vi "Overlay circle modified.vi"(0 "Image In":T1, 1 "Measurment Name":string, 2 "Overlay width":i32, 3 "Overlay color":u32(colorbox), 4 "Circle center":T2, 5 "error in (no error)":errorcluster) -> (14 "Image out":T1, 19 "error out":errorcluster)   [LabVIEW 2019]
uses:
  <vilib>/vision/Image Controls.llb/IMAQ Image.ctl
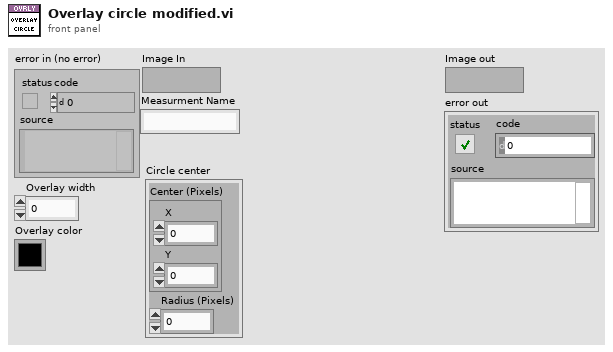
[diagram p1: front panel]
types:
  T1 = typedef "IMAQ Image.ctl" = refnum<image>
  T2 = cluster{"Center (Pixels)":cluster{"X":sgl, "Y":sgl}, "Radius (Pixels)":dbl}
  T3 = cluster{"Left":i32, "Top":i32, "Right":i32, "Bottom":i32}
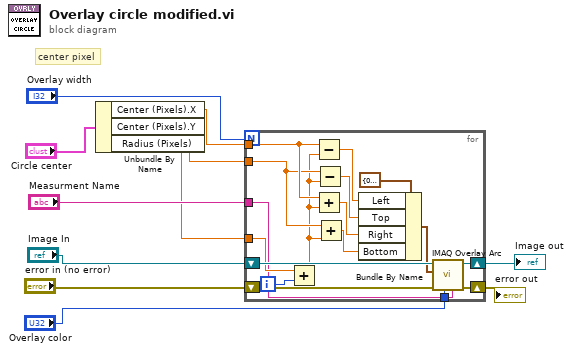
[diagram p0: block diagram]
diagram:
  # "center pixel"
  n1 = Unbundle By Name("Circle center") -> ("Center (Pixels).X"=w4:sgl, "Center (Pixels).Y"=w3:sgl, "Radius (Pixels)"=w2:dbl)
  n2 = for {
    N: "Overlay width" -> [_]
    tunnel: "Overlay color" -> [w24]
    tunnel: w4 -> [w19]
    tunnel: w3 -> [w17]
    tunnel: w2 -> [w14]
    shift-right: [w27] -> w5
    shift-left: "error in (no error)" -> [w28]
    shift-right: [w25] -> w11
    shift-left: "Image In" -> [w26]
    tunnel: "Measurment Name" -> [w12]
    i -> [w15]
    n3 = Add(x=w14, y=w15) -> (x+y=w13:dbl)
    n4 = Subtract(x=w19, y=w13) -> (x-y=w21:dbl)
    n5 = Add(x=w19, y=w13) -> (x+y=w18:dbl)
    n6 = Subtract(x=w17, y=w13) -> (x-y=w20:dbl)
    n7 = Add(x=w17, y=w13) -> (x+y=w16:dbl)
    n8 = Bundle By Name(cluster=T3 {"Left"=0, "Top"=0, "Right"=0, "Bottom"=0} ("Bounding Rectangle"), "Left"=w21, "Top"=w20, "Right"=w18, "Bottom"=w16) -> (w22:T3)
    n9 = call "IMAQ Overlay Arc"("Group"=w12, "Color"=w24, "error in (no error)"=w28, "Bounding Rectangle"=w22, "Image"=w26) -> ("error out"=w27:errorcluster, "Image Out"=w25:T1)  [unwired: 5 in]
  }
  "Image out" <- w11
  "error out" <- w5
